vi "n get status.vi"(8 "error in (no error)":errorcluster, 9 "position":i32, 10 "busy":u16, 11 "n":u16) -> (0 "error out":errorcluster, 1 "position out":i32, 2 "busy out":u16)   [LabVIEW 2015, in "SCANalone4x64.lvlib"]
doc: "__declspec(dllimport) void __stdcall n_get_status(unsigned short n, unsigned short *busy, long *position);"
uses:
  <userlib>/SCANalone4x64/SCANalone4x64.lvlib
  <userlib>/SCANalone4x64/SCANalone4x64.dll
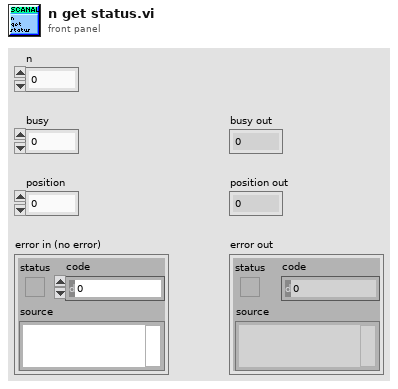
[diagram p1: front panel]
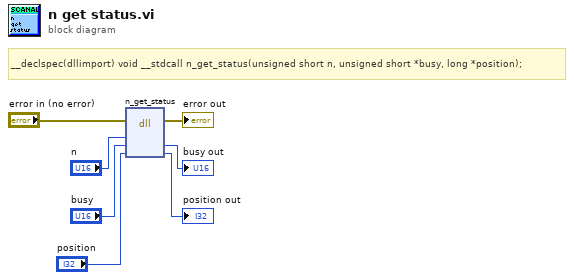
[diagram p0: block diagram]
diagram:
  # "__declspec(dllimport) void __stdcall n_get_status(unsigned short n, unsigned short *busy, long *position);"
  n1 = dll-call lib="C:/Program Files/National Instruments/LabVIEW 2015/user.lib/SCANalone4x64/SCANalone4x64.*" fn="n_get_status"(error in="error in (no error)", "n"="n", "busy"="busy", "position"="position") -> (error out=→"error out":errorcluster, "busy"=→"busy out":u16, "position"=→"position out":i32)  [unwired: 4 in, 1 out]
